vi "sub_joystick_mode-mapping.vi"(9 "joystick info2":T1, 10 "joystick info1":T1, 11 "mode":u8) -> (3 "mode val out":u8)   [LabVIEW 2019]
uses:
  Ctrl/pid-in-params.ctl
  Ctrl/cmd_common.ctl
  Ctrl/gps-databuf.ctl
  Ctrl/sound-data.ctl
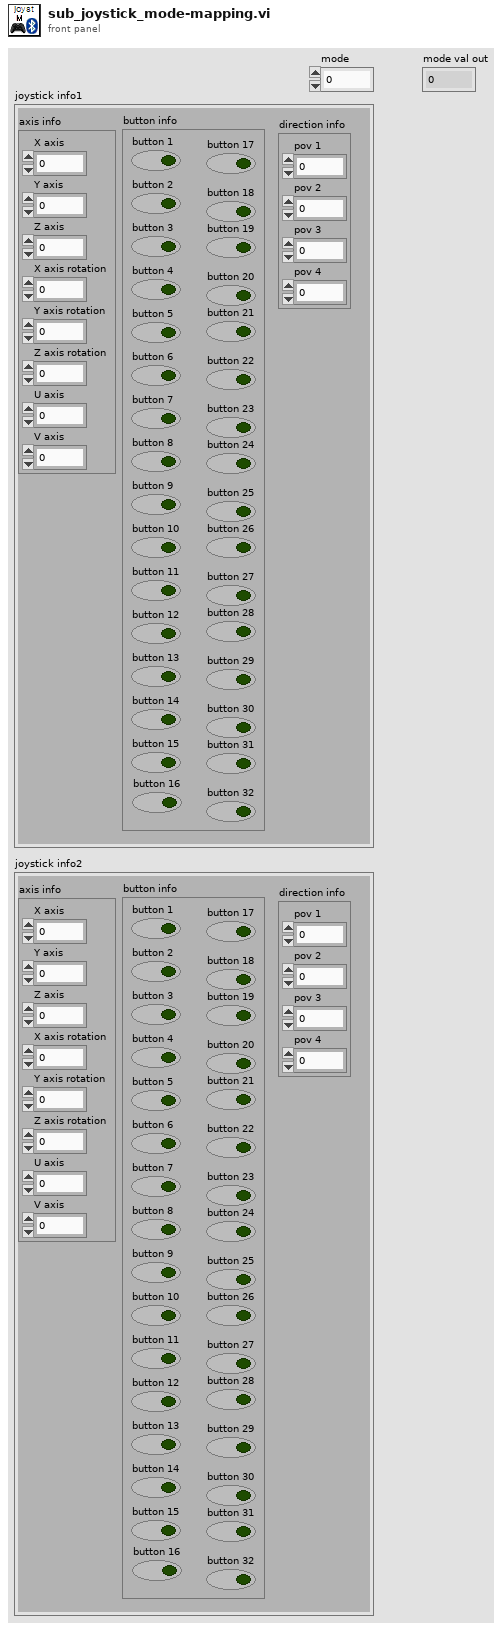
[diagram p1: front panel]
types:
  T1 = cluster{"axis info":cluster{"X axis":i32, "Y axis":i32, "Z axis":i32, "X axis rotation":i32, "Y axis rotation":i32, "Z axis rotation":i32, "U axis":i32, "V axis":i32}, "button info":cluster{"button 1":bool, "button 2":bool, "button 3":bool, "button 4":bool, "button 5":bool, "button 6":bool, "button 7":bool, "button 8":bool, "button 9":bool, "button 10":bool, "button 11":bool, "button 12":bool, "button 13":bool, "button 14":bool, "button 15":bool, "button 16":bool, "button 17":bool, "button 18":bool, "button 19":bool, "button 20":bool, "button 21":bool, "button 22":bool, "button 23":bool, "button 24":bool, "button 25":bool, "button 26":bool, "button 27":bool, "button 28":bool, "button 29":bool, "button 30":bool, "button 31":bool, "button 32":bool}, "direction info":cluster{"pov 1":i32, "pov 2":i32, "pov 3":i32, "pov 4":i32}}
  T2 = cluster{"button 1":bool, "button 2":bool, "button 3":bool, "button 4":bool, "button 5":bool, "button 6":bool, "button 7":bool, "button 8":bool, "button 9":bool, "button 10":bool, "button 11":bool, "button 12":bool, "button 13":bool, "button 14":bool, "button 15":bool, "button 16":bool, "button 17":bool, "button 18":bool, "button 19":bool, "button 20":bool, "button 21":bool, "button 22":bool, "button 23":bool, "button 24":bool, "button 25":bool, "button 26":bool, "button 27":bool, "button 28":bool, "button 29":bool, "button 30":bool, "button 31":bool, "button 32":bool}
  T3 = cluster{"pov 1":i32, "pov 2":i32, "pov 3":i32, "pov 4":i32}
  T4 = typedef "cmd_common.ctl" = enum16{"read", "write"}
  T5 = typedef "sound-data.ctl" = cluster{"FN":enum16{"check", "unlock", "engine", "warning", "msg", "music"}, "Data":variant}
  T6 = enum16{"check", "unlock", "engine", "warning", "msg", "music"}
  T7 = typedef "error_cluster.ctl" = cluster{"AGV":u8, "AGV Estop":u8, "Obstacle":u8, "Heading":u8, "Waypt":u8, "GNSS":u8, "VLP16":u8, "Cam":u8, "RPLidar":u8, "Joystick":u8, "IMU":u8, "Led":u8}
  T8 = typedef "pid-in-params.ctl" = enum16{"read", "write"}
  T9 = typedef "gps-databuf.ctl" = enum16{"read", "write"}
  T10 = cluster{"total time":dbl, "run time":dbl, "wait time":dbl}
  T11 = cluster{"deg_agv-lookahead":dbl, "deg_waypoint":dbl, "deg_gap":dbl, "deg_target":dbl, "pid output":dbl, "dis-gap":dbl, "deg_agv-center":dbl}
  T12 = cluster{"rawdata":string, "GPS Data":cluster{"Latitude":cluster{"Valid?":bool, "Latitude (Deg)":dbl}, "Longitude":cluster{"Valid?":bool, "Longitude (Deg)":dbl}, "Height":cluster{"Valid?":bool, "Height (m)":dbl}, "Undulation":cluster{"Valid?":bool, "Undulation(m)":dbl}, "North Vel":cluster{"Valid?":bool, "North Vel (m/s)":dbl}, "East Vel":cluster{"Valid?":bool, "East Vel (m/s)":dbl}, "Up Vel":cluster{"Valid?":bool, "Up Vel (m/s)":dbl}, "Roll":cluster{"Valid?":bool, "Roll (degrees)":dbl}, "Pitch":cluster{"Valid?":bool, "Pitch (degrees)":dbl}, "Azimuth":cluster{"Valid?":bool, "Azimuth (degrees)":dbl}, "Lat deviation":cluster{"Valid?":bool, "Lat deviation (m)":dbl}, "Long deviation":cluster{"Valid?":bool, "Long deviation (m)":dbl}, "Height deviation":cluster{"Valid?":bool, "Height deviation (m)":dbl}, "North vel deviation":cluster{"Valid?":bool, "North vel deviation (m/s)":dbl}, "East vel deviation":cluster{"Valid?":bool, "East vel deviation (m/s)":dbl}, "Up vel deviation":cluster{"Valid?":bool, "Up vel deviation (m/s)":dbl}, "Roll deviation":cluster{"Valid?":bool, "Roll deviation (degrees)":dbl}, "Pitch deviation":cluster{"Valid?":bool, "Pitch deviation (degrees)":dbl}, "Azimuth deviation":cluster{"Valid?":bool, "Azimuth deviation (degrees)":dbl}, "Ext sol status":cluster{"Valid?":bool, "Ext sol status":dbl}}, "Heading":dbl, "utm-1":cluster{"XN":dbl, "YE":dbl}}
  T13 = typedef "ledmatrix_data.ctl" = cluster{"ip":string, "data":string, "Port":refnum<visa-resource-name>, "time":string}
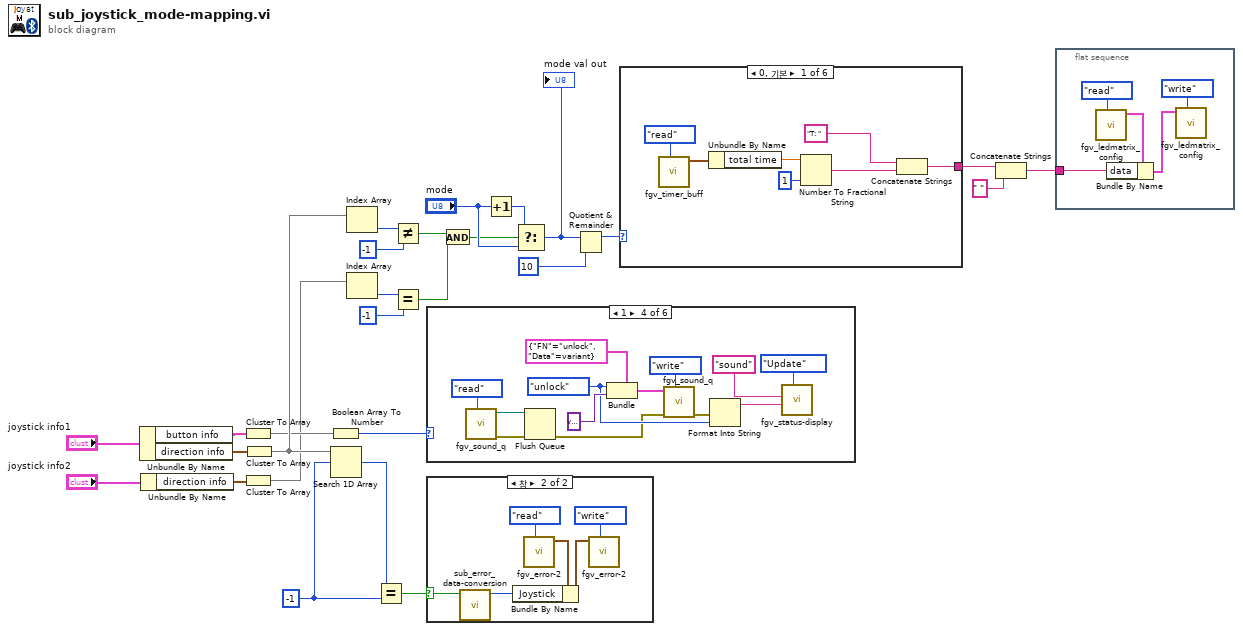
[diagram p0: block diagram]
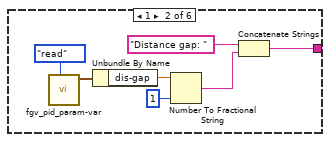
[diagram p2: hidden frame]
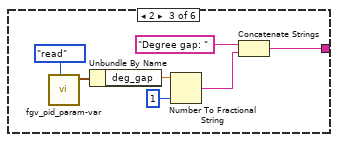
[diagram p3: hidden frame]
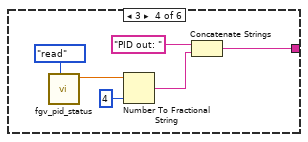
[diagram p4: hidden frame]
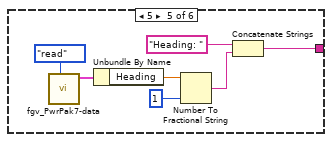
[diagram p5: hidden frame]
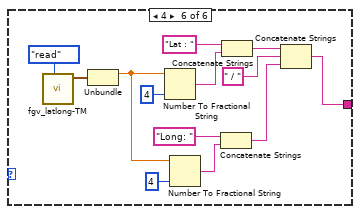
[diagram p6: hidden frame]
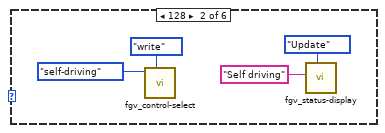
[diagram p8: hidden frame]
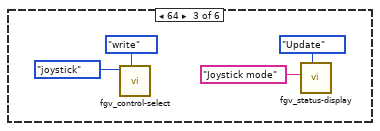
[diagram p9: hidden frame]
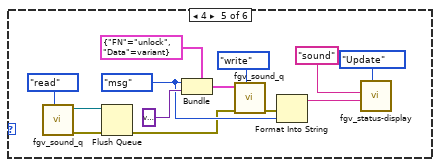
[diagram p10: hidden frame]
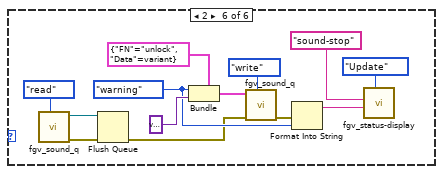
[diagram p11: hidden frame]
diagram:
  w21 = -1 ("element")
  n1 = Unbundle By Name("joystick info1") -> ("button info"=w24:T2, "direction info"=w19:T3)
  n2 = Unbundle By Name("joystick info2") -> ("direction info"=w13:T3)
  n3 = Cluster To Array(cluster=w24) -> (array=w25:bool[])
  n4 = Cluster To Array(cluster=w13) -> (array=w10:i32[])
  n5 = Cluster To Array(cluster=w19) -> (array=w27:i32[])
  n6 = Boolean Array To Number(Boolean array=w25) -> (number=w26:u32)
  n7 = Search 1D Array(1D array=w27, element=w21) -> (index of element=w20:i32)  [unwired: 1 in]
  n8 = Index Array(array=w27) -> (element=w18:i32)  [unwired: 1 in]
  n9 = Index Array(array=w10) -> (element=w11:i32)  [unwired: 1 in]
  n10 = Equal?(x=w20, y=w21) -> (x = y?=w23:bool)
  n11 = Not Equal?(x=w18, y=-1) -> (x != y?=w8:bool)
  n12 = Equal?(x=w11, y=-1) -> (x = y?=w9:bool)
  n13 = case shown="1" w26 {
    frame 0, Default {
    }
    frame 128 {
      n14 = call "fgv_control-select.vi"("cmd"=cmd_common."write", "mode"=enum16{"joystick", "self-driving"}."self-driving") -> ()  [unwired: 9 in, 1 out]
      n15 = call "fgv_status-display.vi"("Mode"=enum16{"Initial", "Update", "Clear"}."Update", "title"="Self driving") -> ()  [unwired: 9 in, 1 out]
    }
    frame 64 {
      n16 = call "fgv_control-select.vi"("cmd"=cmd_common."write", "mode"=enum16{"joystick", "self-driving"}."joystick") -> ()  [unwired: 9 in, 1 out]
      n17 = call "fgv_status-display.vi"("Mode"=enum16{"Initial", "Update", "Clear"}."Update", "title"="Joystick mode") -> ()  [unwired: 9 in, 1 out]
    }
    frame 1 {
      w41 = T6."unlock" ("FN")
      n18 = call "fgv_sound_q.vi"("cmd"=enum16{"create", "write", "read", "close"}."read") -> ("error out"=w38:errorcluster, "queue out"=w37:refnum<queue>)  [unwired: 9 in]
      n19 = Flush Queue(queue=w37, error in (no error)=w38) -> (error out=w36:errorcluster)  [unwired: 2 out]
      n20 = Bundle(cluster=T5 {"FN"=enum."unlock", "Data"=variant} ("data"), "FN"=w41, "Data"=variant) -> (w47:T5)
      n21 = call "fgv_sound_q.vi"("cmd"=enum16{"create", "write", "read", "close"}."write", "error in"=w36, "data"=w47) -> ("error out"=w42:errorcluster)  [unwired: 7 in, 1 out]
      n22 = Format Into String(error in=w42, w41) -> (resulting string=w40:string)  [unwired: 2 in, 1 out]
      n23 = call "fgv_status-display.vi"("Mode"=enum16{"Initial", "Update", "Clear"}."Update", "detail"=w40, "title"="sound") -> ()  [unwired: 8 in, 1 out]
    }
    frame 4 {
      w54 = T6."msg" ("FN")
      n24 = call "fgv_sound_q.vi"("cmd"=enum16{"create", "write", "read", "close"}."read") -> ("error out"=w51:errorcluster, "queue out"=w50:refnum<queue>)  [unwired: 9 in]
      n25 = Flush Queue(queue=w50, error in (no error)=w51) -> (error out=w49:errorcluster)  [unwired: 2 out]
      n26 = Bundle(cluster=T5 {"FN"=enum."unlock", "Data"=variant} ("data"), "FN"=w54, "Data"=variant) -> (w60:T5)
      n27 = call "fgv_sound_q.vi"("cmd"=enum16{"create", "write", "read", "close"}."write", "error in"=w49, "data"=w60) -> ("error out"=w55:errorcluster)  [unwired: 7 in, 1 out]
      n28 = Format Into String(error in=w55, w54) -> (resulting string=w53:string)  [unwired: 2 in, 1 out]
      n29 = call "fgv_status-display.vi"("Mode"=enum16{"Initial", "Update", "Clear"}."Update", "detail"=w53, "title"="sound") -> ()  [unwired: 8 in, 1 out]
    }
    frame 2 {
      w67 = T6."warning" ("FN")
      n30 = call "fgv_sound_q.vi"("cmd"=enum16{"create", "write", "read", "close"}."read") -> ("error out"=w64:errorcluster, "queue out"=w63:refnum<queue>)  [unwired: 9 in]
      n31 = Flush Queue(queue=w63, error in (no error)=w64) -> (error out=w62:errorcluster)  [unwired: 2 out]
      n32 = Bundle(cluster=T5 {"FN"=enum."unlock", "Data"=variant} ("data"), "FN"=w67, "Data"=variant) -> (w73:T5)
      n33 = call "fgv_sound_q.vi"("cmd"=enum16{"create", "write", "read", "close"}."write", "error in"=w62, "data"=w73) -> ("error out"=w68:errorcluster)  [unwired: 7 in, 1 out]
      n34 = Format Into String(error in=w68, w67) -> (resulting string=w66:string)  [unwired: 2 in, 1 out]
      n35 = call "fgv_status-display.vi"("Mode"=enum16{"Initial", "Update", "Clear"}."Update", "detail"=w66, "title"="sound-stop") -> ()  [unwired: 8 in, 1 out]
    }
  }
  n36 = case shown="참" w23 {
    selector: w23 -> [_ w75]
    frame False {
    }
    frame True {
      n37 = call "sub_error_data-conversion.vi"("error status"=w75) -> ("error conversion out"=w78:u8)  [unwired: 9 in, 1 out]
      n38 = call "fgv_error-2.vi"("cmd"=enum16{"init", "read", "write"}."read") -> ("Error cluster out"=w77:T7)  [unwired: 9 in, 1 out]
      n39 = Bundle By Name(cluster=w77, "Joystick"=w78) -> (w76:T7)
      n40 = call "fgv_error-2.vi"("cmd"=enum16{"init", "read", "write"}."write", "Error cluster"=w76) -> ()  [unwired: 8 in, 2 out]
    }
  }
  n41 = And(x=w8, y=w9) -> (x .and. y?=w7:bool)
  n42 = Increment(x="mode") -> (x+1=w16:u8)
  n43 = Select(t=w16, s=w7, f="mode") -> (s? t:f=w6:u8)
  "mode val out" <- w6
  n44 = Quotient & Remainder(x=w6, y=u8 10) -> (x-y*floor(x/y)=w4:u8)  [unwired: 1 out]
  n45 = case shown="0, 기본" w4 {
    tunnel: [w81 w88 w95 w104 w111 w119] -> w3
    frame 0, Default {
      n46 = call "fgv_timer_buff.vi"("cmd"=enum16{"write", "read"}."read") -> ("time_status out"=w86:T10)  [unwired: 10 in]
      n47 = Unbundle By Name(w86) -> ("total time"=w85:dbl)
      n48 = Number To Fractional String(number=w85, precision (6)=i16 1 ("정밀도(6)")) -> (F-format string=w83:string)  [unwired: 2 in]
      n49 = Concatenate Strings("T: ", w83) -> (w81:string)
    }
    frame 1 {
      n50 = call "fgv_pid_param-var.vi"("cmd"=pid-in-params."read") -> ("pid-var_output"=w93:T11)  [unwired: 10 in]
      n51 = Unbundle By Name(w93) -> ("dis-gap"=w91:dbl)
      n52 = Number To Fractional String(number=w91, precision (6)=i16 1 ("정밀도(6)")) -> (F-format string=w89:string)  [unwired: 2 in]
      n53 = Concatenate Strings("Distance gap: " ("문자열"), w89) -> (w88:string)
    }
    frame 2 {
      n54 = call "fgv_pid_param-var.vi"("cmd"=pid-in-params."read") -> ("pid-var_output"=w100:T11)  [unwired: 10 in]
      n55 = Unbundle By Name(w100) -> ("deg_gap"=w98:dbl)
      n56 = Number To Fractional String(number=w98, precision (6)=i16 1 ("정밀도(6)")) -> (F-format string=w96:string)  [unwired: 2 in]
      n57 = Concatenate Strings("Degree gap: " ("문자열"), w96) -> (w95:string)
    }
    frame 3 {
      n58 = call "fgv_pid_status.vi"("cmd"=cmd_common."read") -> ("pid output"=w102:dbl)  [unwired: 8 in, 2 out]
      n59 = Number To Fractional String(number=w102, precision (6)=i16 4 ("정밀도(6)")) -> (F-format string=w105:string)  [unwired: 2 in]
      n60 = Concatenate Strings("PID out: " ("문자열"), w105) -> (w104:string)
    }
    frame 5 {
      n61 = call "fgv_PwrPak7-data.vi"("cmd"=gps-databuf."read") -> ("data cluster out"=w109:T12)  [unwired: 9 in, 1 out]
      n62 = Unbundle By Name(w109) -> ("Heading"=w108:dbl)
      n63 = Number To Fractional String(number=w108, precision (6)=i16 1 ("정밀도(6)")) -> (F-format string=w112:string)  [unwired: 2 in]
      n64 = Concatenate Strings("Heading: " ("문자열"), w112) -> (w111:string)
    }
    frame 4 {
      n65 = call "fgv_latlong-TM.vi"("cmd"=enum16{"write", "read"}."read") -> ("latlong out"=w122:cluster{"lat":dbl, "long":dbl})  [unwired: 9 in, 1 out]
      n66 = Unbundle(w122) -> ("lat"=w116:dbl)  [unwired: 1 out]
      n67 = Number To Fractional String(number=w116, precision (6)=i16 4 ("정밀도(6)")) -> (F-format string=w125:string)  [unwired: 2 in]
      n68 = Number To Fractional String(number=w116, precision (6)=i16 4 ("정밀도(6)")) -> (F-format string=w117:string)  [unwired: 2 in]
      n69 = Concatenate Strings("Long: " ("문자열"), w117) -> (w121:string)
      n70 = Concatenate Strings("Lat : " ("문자열"), w125) -> (w120:string)
      n71 = Concatenate Strings(w120, " / " ("문자열"), w121) -> (w119:string)
    }
  }
  n72 = Concatenate Strings(w3, " " ("문자열")) -> (w1:string)
  n73 = flat-sequence {
    tunnel: w1 -> [w128]
    frame #0 {
      n74 = call "fgv_ledmatrix_config.vi"("cmd"=cmd_common."read") -> ("data out"=w130:T13)  [unwired: 10 in]
      n75 = Bundle By Name(cluster=w130, "data"=w128) -> (w129:T13)
      n76 = call "fgv_ledmatrix_config.vi"("cmd"=cmd_common."write", "data"=w129) -> ()  [unwired: 9 in, 1 out]
    }
  }
